vi "Prepare Status Table.vi"(7 "MulticolumnListbox in":refnum<vi>, 9 "Temp:UploadingFile":path, 10 "Upload List":path[](array[path])) -> (2 "Array":string[][](array[string]))   [LabVIEW 2020]
uses:
  <vilib>/Utility/miscctls.llb/LVRowAndColumnTypeDef.ctl
  <userlib>/_NEVSTOP/Communicable State Machine(CSM)/Communicable State Machine.lvlib
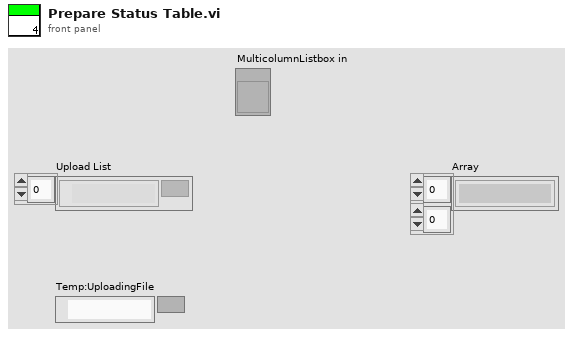
[diagram p1: front panel]
types:
  T1 = typedef "LVRowAndColumnTypeDef.ctl" = cluster{"Row":i32, "Column":i32}
  T2 = cluster{"Font Name:":string, "Size":i16, "Strikeout?":bool, "Italic?":bool, "Underline?":bool, "Outline?":bool, "Shadow?":bool, "Bold?":bool}
  T3 = typedef "LVFontTypeDef.ctl" = cluster{"Font Name":string, "Size":u16, "Bold":bool, "Italic":bool, "Underline":bool, "Strikeout":bool, "Color":u32}
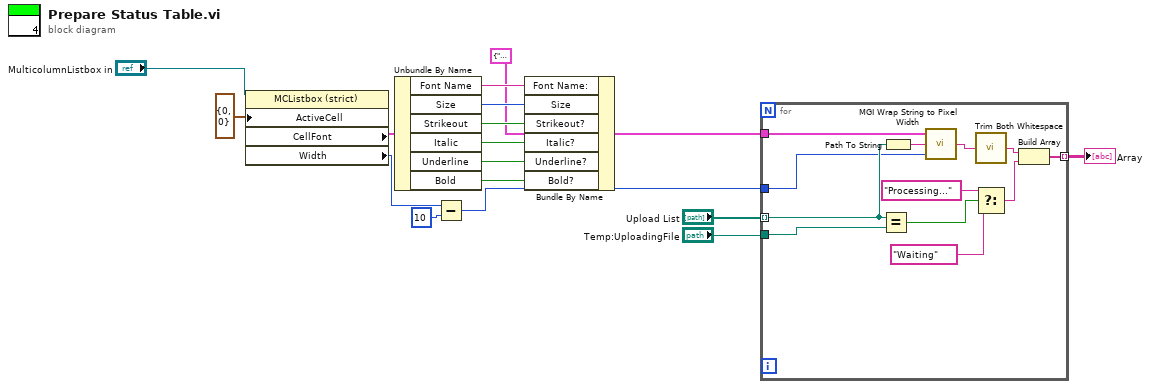
[diagram p0: block diagram]
diagram:
  n1 = property on="Property Node" class="MCListbox (strict)"(reference="MulticolumnListbox in", "ActiveCell"=T1 {"Row"=0, "Column"=0} ("Active Cell:Active Cell")) -> ("CellFont"=w13:T3, "Width"=w15:u32)  [unwired: 1 in, 2 out]
  n2 = Unbundle By Name(w13) -> ("Font Name"=w7:string, "Size"=w12:u16, "Strikeout"=w11:bool, "Italic"=w10:bool, "Underline"=w9:bool, "Bold"=w8:bool)
  n3 = Subtract(x=w15, y=u32 10) -> (x-y=w14:u32)
  n4 = Bundle By Name(cluster=T2 {"Font Name:"="", "Size"=0, "Strikeout?"=FALSE, "Italic?"=FALSE, "Underline?"=FALSE, "Outline?"=FALSE, "Shadow?"=FALSE, "Bold?"=FALSE} ("Font"), "Font Name:"=w7, "Size"=w12, "Strikeout?"=w11, "Italic?"=w10, "Underline?"=w9, "Bold?"=w8) -> (w6:T2)
  n5 = for {
    tunnel: "Upload List" -> [w24] mode=indexing
    tunnel: [w28] -> w3 mode=indexing
    tunnel: "Temp:UploadingFile" -> [w23]
    tunnel: w14 -> [w20]
    tunnel: w6 -> [w19]
    n6 = Equal?(x=w24, y=w23) -> (x = y?=w25:bool)
    n7 = Path To String(path=w24) -> (string=w22:string)
    n8 = call <userlib>:"MGI Wrap String to Pixel Width.vi"("Width"=w20, "String"=w22, "Font"=w19) -> ("Wrapped String"=w21:string)
    n9 = call <userlib>:"Trim Both Whitespace.vi"("string"=w21) -> ("trimmed string"=w18:string)  [unwired: 1 in]
    n10 = Select(t="Processing...", s=w25, f="Waiting") -> (s? t:f=w29:string)
    n11 = Build Array(w18, w29) -> (w28:string[])
  }
  "Array" <- w3
